vi "环动报警队列存储.vi"() -> ()   [LabVIEW 2016, in "环境动力监测库.lvlib"]
uses:
  <vilib>/addons/database/Auxilliary.llb/DB Tools Column Info.ctl
  <vilib>/addons/database/Auxilliary.llb/DB Tools DataTypes.ctl
  <vilib>/addons/database/NI_Database_API.lvlib
  <vilib>/Utility/VariantDataType/VariantType.lvlib
panel:
  in  "data in":T1
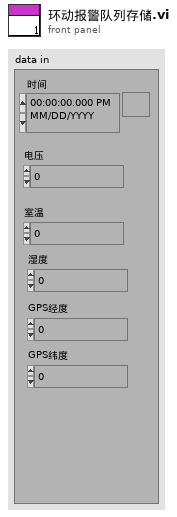
[diagram p1: front panel]
types:
  T1 = cluster{"时间":timestamp, "电压":dbl, "室温":dbl, "湿度":dbl, "GPS经度":dbl, "GPS纬度":dbl}
  T2 = typedef "NI_Database_API.lvlib/DB Tools Column Info.ctl" = cluster{"column name":string, "data type":T3, "size":i32, "allow null?":bool}
  T3 = typedef "NI_Database_API.lvlib/DB Tools DataTypes.ctl" = enum16{"String", "Long (I32)", "Single (SGL)", "Double (DBL)", "Date/Time", "Binary"}
  T4 = cluster{"市电监测":bool, "用水量监测":bool, "烟雾监测":bool, "温度湿度":bool, "振动监测":bool, "红外入侵监测":bool, "漏水监测":bool, "门禁开关监测":bool, "视频监测":bool, "UPS监测":bool, "空调监测":bool, "冰箱监测":bool, "排气扇监测":bool, "蓄电池监测":bool, "GPS监测":bool, "北斗监测":bool, "气象监测":bool}
  T5 = cluster{"传感器":cluster{"红外监测":bool, "振动监测":bool, "烟雾监测":bool, "门禁监测":bool, "水浸监测":bool}, "北斗-GPS":cluster{"北斗":cluster{"北斗经度:":sgl, "北斗纬度:":sgl}, "GPS":cluster{"GPS经度: ":sgl, "GPS纬度: ":sgl}}, "气象仪":cluster{"气温: ":sgl, "气压: ":sgl, "风速:":sgl, "风向:":sgl, "气象仪经度: ":sgl, "气象仪纬度: ":sgl}}
  T6 = cluster{"市电":cluster{"电压:":u16, "电流：":dbl, "状态":bool}, "UPS":cluster{"输入电压:":sgl, "输出电压:":sgl, "电池电量:":u8, "电量":u16, "状态":bool}, "蓄电池":cluster{"电压:":sgl, "电流:":sgl, "电池电量:":u8, "电量":u16, "状态":bool}}
  T7 = cluster{"温湿度":cluster{"温度:":sgl, "状态":bool, "湿度:":sgl}, "空调":cluster{"机柜温度:":sgl, "状态":bool, "压缩机:":enum16{"停止", "运行"}, "电加热:":enum16{"停止", "运行"}}, "排气扇":cluster{"排气扇:":enum16{"关闭", "打开"}}, "冰箱":cluster{"冰箱:":enum16{"关闭", "打开"}}}
  T8 = typedef "LVDateTimeRec.ctl" = cluster{"秒数的小数部分":dbl, "秒":i32, "分":i32, "时":i32, "日":i32, "月":i32, "年":i32, "天数（周）":i32, "天数（年）":i32, "DST":i32}
  T9 = typedef "VariantType.lvlib/Type.ctl" = enum8{"Invalid Type", "Void", "I8", "I16", "I32", "I64", "U8", "U16", "U32", "U64", "Single Float", "Double Float", "Extended Float", "Single Complex", "Double Complex", "Extended Complex", "Enum U8", "Enum U16", "Enum U32", "Enum U64", "Single Float With Unit", "Double Float With Unit", "Extended Float With Unit", "Single Complex with Unit", "Double Complex with Unit", "Extended Complex with Unit", "Boolean", "String", "Path", "Picture", "Tag", "Array", "Cluster", "Variant", "LV Variant", "Waveform", "Timestamp", "Digital Waveform", "Digital Data", "ExpressData", "Refnum", "External Data", "VI", "Poly VI", "LabVIEW Class Instance", "Fixed Point"}
  T10 = cluster{"时间标识":timestamp, "设备":string, "日志信息":string}
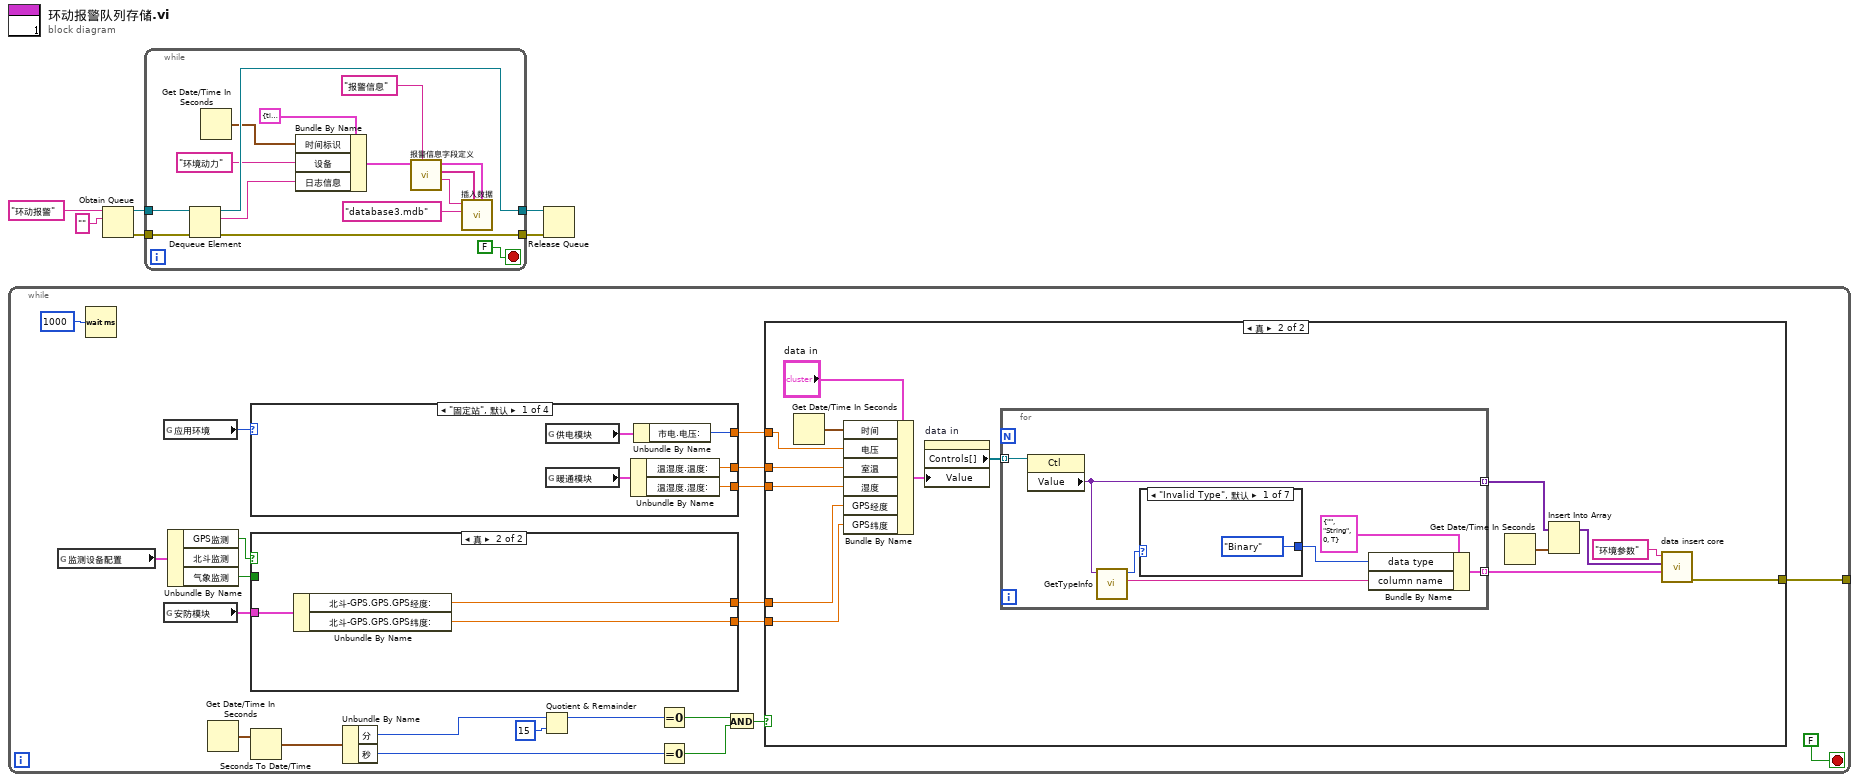
[diagram p0: block diagram]
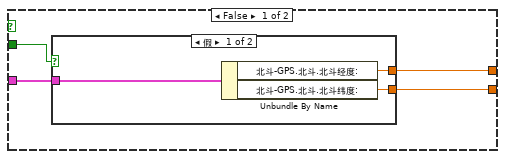
[diagram p2: hidden frame]
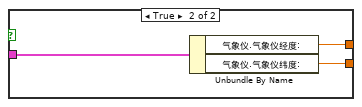
[diagram p3: hidden frame]
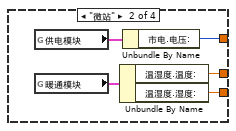
[diagram p4: hidden frame]
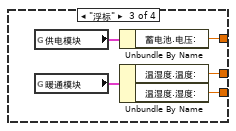
[diagram p5: hidden frame]
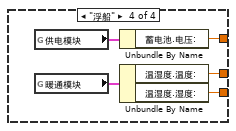
[diagram p6: hidden frame]
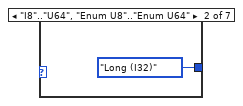
[diagram p8: hidden frame]
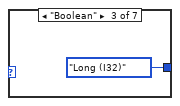
[diagram p9: hidden frame]
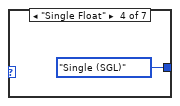
[diagram p10: hidden frame]
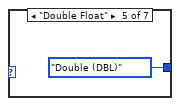
[diagram p11: hidden frame]
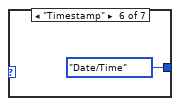
[diagram p12: hidden frame]
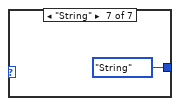
[diagram p13: hidden frame]
diagram:
  n1 = while {
    tunnel: [w26] -> _
    stop <- FALSE stop-if-true
    n2 = global read "断电保存全局变量.vi" "监测设备配置"() -> (w12:T4)
    n3 = Wait (ms)(milliseconds to wait=u32 1000 ("等待时间（毫秒）")) -> ()  [unwired: 1 out]
    n4 = global read "外部交互全局变量.vi" "应用环境"() -> (w16:enum16{"固定站", "微站", "浮标", "浮船"})
    n5 = global read "内部交互全局变量.vi" "安防模块"() -> (w10:T5)
    n6 = Unbundle By Name(w12) -> ("GPS监测"=w11:bool, "气象监测"=w7:bool)  [unwired: 1 out]
    n7 = Get Date/Time In Seconds() -> (seconds since 1Jan1904=w25:timestamp)
    n8 = case shown="\"固定站\", 默认" w16 {
      tunnel: [w45 w49 w54 w59] -> w15
      tunnel: [w43 w48 w53 w58] -> w14
      tunnel: [w42 w47 w52 w57] -> w13
      frame "固定站", Default {
        n9 = global read "内部交互全局变量.vi" "供电模块"() -> (w46:T6)
        n10 = global read "内部交互全局变量.vi" "暖通模块"() -> (w44:T7)
        n11 = Unbundle By Name(w44) -> ("温湿度.温度:"=w43:sgl, "温湿度.湿度:"=w42:sgl)
        n12 = Unbundle By Name(w46) -> ("市电.电压:"=w45:u16)
      }
      frame "微站" {
        n13 = global read "内部交互全局变量.vi" "供电模块"() -> (w51:T6)
        n14 = global read "内部交互全局变量.vi" "暖通模块"() -> (w50:T7)
        n15 = Unbundle By Name(w50) -> ("温湿度.温度:"=w48:sgl, "温湿度.湿度:"=w47:sgl)
        n16 = Unbundle By Name(w51) -> ("市电.电压:"=w49:u16)
      }
      frame "浮标" {
        n17 = global read "内部交互全局变量.vi" "供电模块"() -> (w56:T6)
        n18 = global read "内部交互全局变量.vi" "暖通模块"() -> (w55:T7)
        n19 = Unbundle By Name(w56) -> ("蓄电池.电压:"=w54:sgl)
        n20 = Unbundle By Name(w55) -> ("温湿度.温度:"=w53:sgl, "温湿度.湿度:"=w52:sgl)
      }
      frame "浮船" {
        n21 = global read "内部交互全局变量.vi" "供电模块"() -> (w61:T6)
        n22 = global read "内部交互全局变量.vi" "暖通模块"() -> (w60:T7)
        n23 = Unbundle By Name(w61) -> ("蓄电池.电压:"=w59:sgl)
        n24 = Unbundle By Name(w60) -> ("温湿度.温度:"=w58:sgl, "温湿度.湿度:"=w57:sgl)
      }
    }
    n25 = case shown="真" w11 {
      tunnel: w10 -> [w31 w41]
      tunnel: [w30 w40] -> w9
      tunnel: [w29 w39] -> w8
      tunnel: w7 -> [w32 _]
      frame False {
        n26 = case shown="假" w32 {
          tunnel: w31 -> [w33 w38]
          tunnel: [w35 w37] -> w30
          tunnel: [w34 w36] -> w29
          frame False {
            n27 = Unbundle By Name(w33) -> ("北斗-GPS.北斗.北斗经度:"=w35:sgl, "北斗-GPS.北斗.北斗纬度:"=w34:sgl)
          }
          frame True {
            n28 = Unbundle By Name(w38) -> ("气象仪.气象仪经度:"=w37:sgl, "气象仪.气象仪纬度:"=w36:sgl)
          }
        }
      }
      frame True {
        n29 = Unbundle By Name(w41) -> ("北斗-GPS.GPS.GPS经度:"=w40:sgl, "北斗-GPS.GPS.GPS纬度:"=w39:sgl)
      }
    }
    n30 = Seconds To Date/Time(time stamp (now)=w25) -> (date time rec=w18:T8)  [unwired: 1 in]
    n31 = Unbundle By Name(w18) -> ("分"=w19:i32, "秒"=w22:i32)
    n32 = Quotient & Remainder(x=w19, y=15) -> (x-y*floor(x/y)=w21:i32)  [unwired: 1 out]
    n33 = Equal To 0?(x=w21) -> (x = 0?=w23:bool)
    n34 = Equal To 0?(x=w22) -> (x = 0?=w24:bool)
    n35 = And(x=w23, y=w24) -> (x .and. y?=w17:bool)
    n36 = case shown="真" w17 {
      tunnel: [_ w67] -> w26
      tunnel: w15 -> [_ w66]
      tunnel: w14 -> [_ w65]
      tunnel: w13 -> [_ w64]
      tunnel: w9 -> [_ w63]
      tunnel: w8 -> [_ w62]
      frame False {
      }
      frame True {
        n37 = Get Date/Time In Seconds() -> (seconds since 1Jan1904=w69:timestamp)
        n38 = Bundle By Name(cluster="data in", "时间"=w69, "电压"=w66, "室温"=w65, "湿度"=w64, "GPS经度"=w63, "GPS纬度"=w62) -> (w68:T1)
        n39 = property on="data in" class="Clust (严格)"("Value"=w68) -> ("Controls[]"=w71:refnum<vi>[])  [unwired: 2 in, 2 out]
        n40 = for {
          tunnel: w71 -> [w83] mode=indexing
          tunnel: [w77] -> w76 mode=indexing
          tunnel: [w78] -> w73 mode=indexing
          n41 = property class="Ctl"(reference=w83) -> ("Value"=w77:variant)  [unwired: 1 in, 2 out]
          n42 = call <vilib>:"GetTypeInfo.vi"("Variant"=w77) -> ("Name"=w81:string, "Type Enum"=w80:T9)  [unwired: 6 in, 3 out]
          n43 = case shown="\"Invalid Type\", 默认" w80 {
            tunnel: [DB_Tools_DataTypes."Binary" ("data type") DB_Tools_DataTypes."Long (I32)" ("data type") DB_Tools_DataTypes."Long (I32)" ("data type") DB_Tools_DataTypes."Single (SGL)" ("data type") DB_Tools_DataTypes."Double (DBL)" ("data type") DB_Tools_DataTypes."Date/Time" ("data type") DB_Tools_DataTypes."String" ("data type")] -> w79
            frame "Invalid Type", Default {
            }
            frame "I8".."U64", "Enum U8".."Enum U64" {
            }
            frame "Boolean" {
            }
            frame "Single Float" {
            }
            frame "Double Float" {
            }
            frame "Timestamp" {
            }
            frame "String" {
            }
          }
          n44 = Bundle By Name(cluster=T2 {"column name"="", "data type"=enum."String", "size"=0, "allow null?"=TRUE} ("column information"), "data type"=w79, "column name"=w81) -> (w78:T2)
        }
        n45 = Get Date/Time In Seconds() -> (seconds since 1Jan1904=w75:timestamp)
        n46 = Insert Into Array(array=w76, new element=w75) -> (w74:variant[])  [unwired: 1 in]
        n47 = call "data insert core.vi"("column information"=w73, "data"=w74, "table"="环境参数") -> ("error out"=w67:errorcluster)  [unwired: 8 in]
      }
    }
  }
  n48 = Obtain Queue(name (unnamed)="环动报警" ("名称（未命名）"), element data type="" ("报警内容")) -> (queue out=w6:refnum<queue>, error out=w5:errorcluster)  [unwired: 3 in, 1 out]
  n49 = while {
    tunnel: w6 -> [w105]
    tunnel: w5 -> [w104]
    tunnel: [w102] -> w3
    tunnel: [w101] -> w2
    stop <- FALSE stop-if-true
    n50 = Dequeue Element(queue=w105, error in (no error)=w104) -> (queue out=w102:refnum<queue>, element=w91:string, error out=w101:errorcluster)  [unwired: 1 in, 1 out]
    n51 = Get Date/Time In Seconds() -> (seconds since 1Jan1904=w93:timestamp)
    n52 = Bundle By Name(cluster=T10 {"时间标识"=timestamp(0 s since 1904-01-01), "设备"="", "日志信息"=""} ("data in"), "时间标识"=w93, "设备"="环境动力", "日志信息"=w91) -> (w94:T10)
    n53 = call "报警信息字段定义.vi"("table输入"="报警信息", "data in"=w94) -> ("table输出"=w98:string, "columns"=w99:string[], "data out"=w100:T10)  [unwired: 7 in]
    n54 = call "插入数据.vi"("data"=w100, "columns"=w99, "database"="database3.mdb", "table"=w98) -> ()  [unwired: 7 in, 1 out]
  }
  n55 = Release Queue(queue=w3, error in (no error)=w2) -> ()  [unwired: 1 in, 3 out]
